vi "InitConstantsPerformReset.vi"   [LabVIEW 2019]
doc: "This VI sets constants and resets the global variables."
uses:
  constants.vi
  outputs.vi
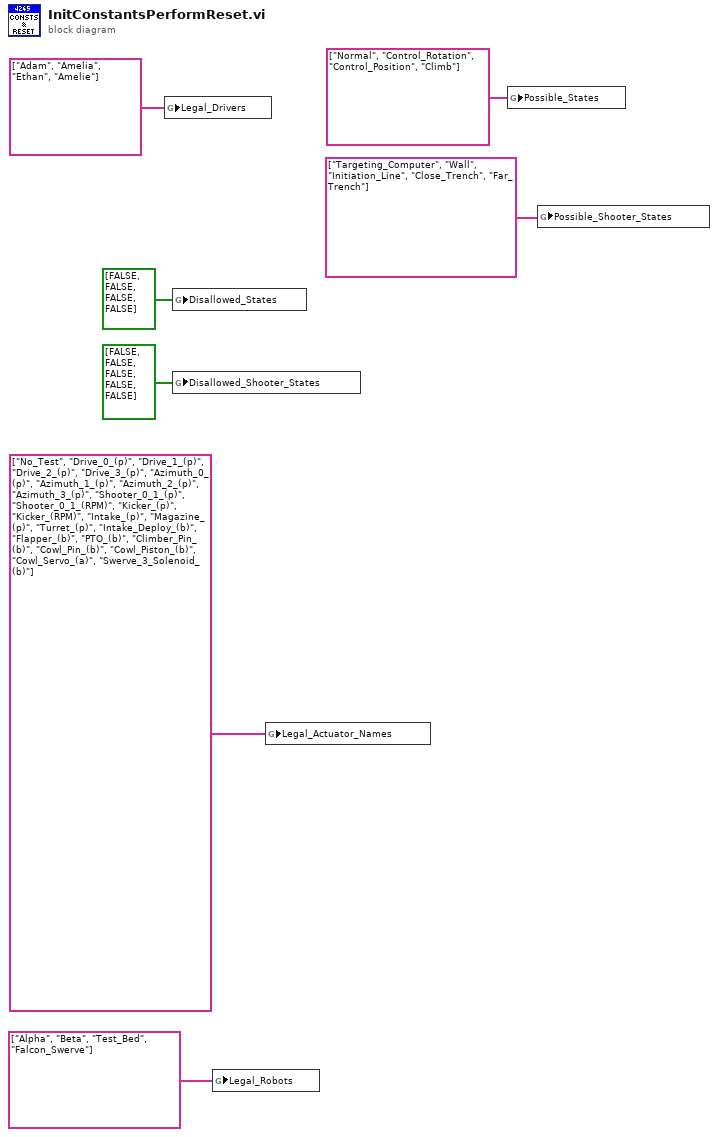
[diagram p0: block diagram]
diagram:
  n1 = global write "constants.vi" "Legal_Drivers"(string[] ["Adam", "Amelia", "Ethan", "Amelie"] ("appended array")) -> ()
  n2 = global write "outputs.vi" "Disallowed_States"(bool[] [FALSE, FALSE, FALSE, FALSE] ("appended array")) -> ()
  n3 = global write "outputs.vi" "Disallowed_Shooter_States"(bool[] [FALSE, FALSE, FALSE, FALSE, FALSE] ("appended array")) -> ()
  n4 = global write "constants.vi" "Legal_Robots"(string[] ["Alpha", "Beta", "Test_Bed", "Falcon_Swerve"] ("Legal_Actuator_Names")) -> ()
  n5 = global write "constants.vi" "Legal_Actuator_Names"(string[] ["No_Test", "Drive_0_(p)", "Drive_1_(p)", "Drive_2_(p)", "Drive_3_(p)", "Azimuth_0_(p)", "Azimuth_1_(p)", "Azimuth_2_(p)", "Azimuth_3_(p)", "Shooter_0_1_(p)", "Shooter_0_1_(RPM)", "Kicker_(p)", "Kicker_(RPM)", "Intake_(p)", "Magazine_(p)", "Turret_(p)", "Intake_Deploy_(b)", "Flapper_(b)", "PTO_(b)", "Climber_Pin_(b)", "Cowl_Pin_(b)", "Cowl_Piston_(b)", "Cowl_Servo_(a)", "Swerve_3_Solenoid_(b)"] ("appended array")) -> ()
  n6 = global write "constants.vi" "Possible_States"(string[] ["Normal", "Control_Rotation", "Control_Position", "Climb"] ("appended array")) -> ()
  n7 = global write "constants.vi" "Possible_Shooter_States"(string[] ["Targeting_Computer", "Wall", "Initiation_Line", "Close_Trench", "Far_Trench"] ("appended array")) -> ()
